vi "Resolve Template Value.vi"(6 "Locals":refnum<class "Value Tree.lvclass">, 7 "Folder":path, 8 "error in (no error)":errorcluster, 9 "Template Service in":refnum<class "TemplateService.lvclass">, 10 "Value Name":string, 11 "VolatusVariableResolver in":refnum<class "VolatusVariableResolver.lvclass">) -> (0 "error out":errorcluster, 1 "Template Service":refnum<class "TemplateService.lvclass">, 2 "Value":refnum<class "Value Tree.lvclass">)   [LabVIEW 2020, in "Volatus.lvlib" / "VolatusVariableResolver.lvclass"]
uses:
  VolatusVariableResolver.lvclass
  VolatusVariableResolver.lvclass/VolatusVariableResolver.ctl
  VolatusAPI/VolatusAPI.lvclass
  lv-http-server/HTTP Server/Value Tree/Value Tree.lvclass
  lv-http-server/HTTP Server/TemplateService/TemplateService.lvclass
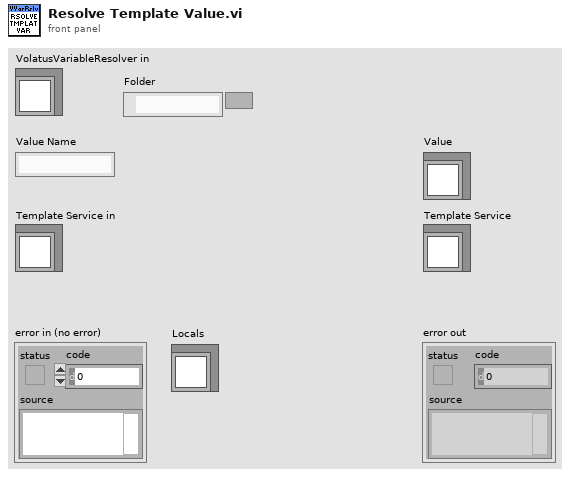
[diagram p1: front panel]
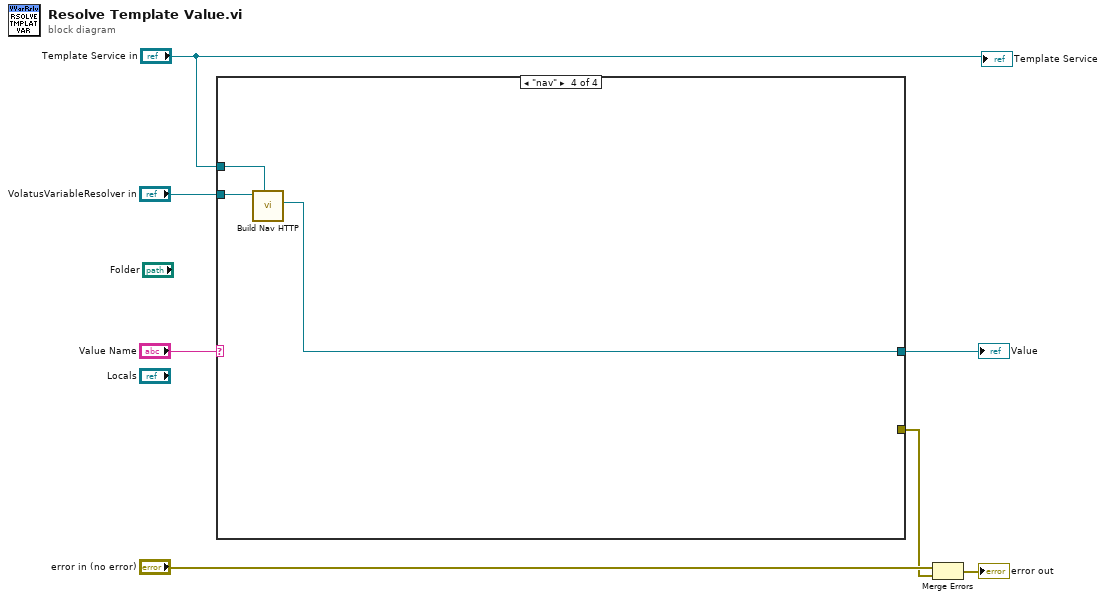
[diagram p0: block diagram]
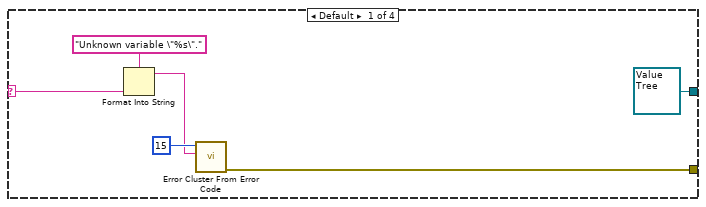
[diagram p2: hidden frame]
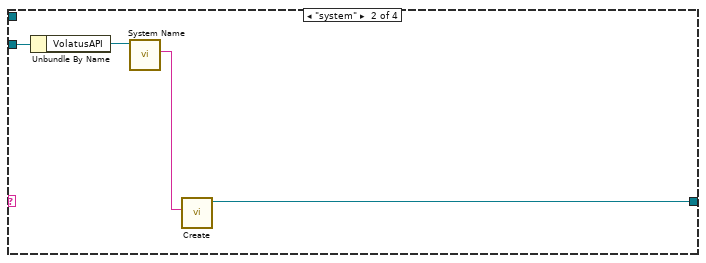
[diagram p3: hidden frame]
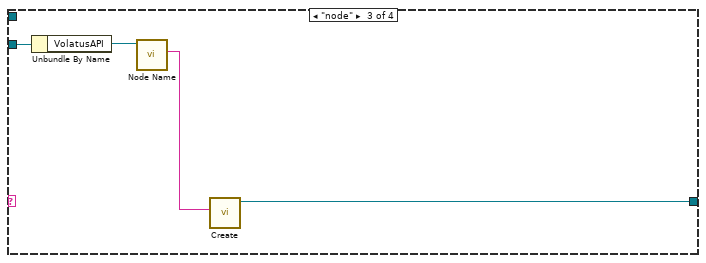
[diagram p4: hidden frame]
diagram:
  n1 = case shown="\"nav\"" "Value Name" {
    selector: "Value Name" -> [w12 _ _ _]
    tunnel: "VolatusVariableResolver in" -> [_ w17 w21 w24]
    tunnel: [refnum<class "Value Tree.lvclass"> refnum ("Value Tree out") w14 w18 w22] -> w4
    tunnel: [w9 _ _ _] -> w2
    tunnel: "Template Service in" -> [_ _ _ w23]
    frame Default {
      n2 = Format Into String(format string="Unknown variable \"%s\".", w12) -> (resulting string=w10:string)  [unwired: 2 in, 1 out]
      n3 = call <vilib>:"Error Cluster From Error Code.vi"("error message (\"\")"=w10, "error code (0)"=15) -> ("error out"=w9:errorcluster)  [unwired: 7 in]
    }
    frame "system" {
      n4 = Unbundle By Name(w17) -> ("VolatusAPI"=w16:refnum<class "VolatusAPI.lvclass">)
      n5 = call "System Name.vi"("VolatusAPI in"=w16) -> ("System"=w15:string)  [unwired: 9 in, 1 out]
      n6 = call "Create.vi"("Value"=w15) -> ("Value Tree out"=w14:refnum<class "Value Tree.lvclass">)  [unwired: 10 in]
    }
    frame "node" {
      n7 = Unbundle By Name(w21) -> ("VolatusAPI"=w20:refnum<class "VolatusAPI.lvclass">)
      n8 = call "Node Name.vi"("VolatusAPI in"=w20) -> ("Node Name"=w19:string)  [unwired: 8 in, 2 out]
      n9 = call "Create.vi"("Value"=w19) -> ("Value Tree out"=w18:refnum<class "Value Tree.lvclass">)  [unwired: 10 in]
    }
    frame "nav" {
      n10 = call "Build Nav HTTP.vi"("TemplateService"=w23, "VolatusVariableResolver in"=w24) -> ("Value"=w22:refnum<class "Value Tree.lvclass">)  [unwired: 9 in]
    }
  }
  "Value" <- w4
  n11 = Merge Errors("error in (no error)", w2) -> (→"error out":errorcluster)
  "Template Service" <- "Template Service in"
